vi "CTRE_PigeonIMU_GetYPR.vi"(8 "error in (no error)":errorcluster, 11 "PigeonIMUDevRef":T1={"DeviceStatus"={"status"=FALSE, "code"=0, "source"=""}, "Device Number"=0, "Type"=352321536, "Device ID"=0, "Handle"=0, "UsageFrame"=0, "Library Path"=path ""} {"Type" items=["CAN"=352321536, "TalonSRX"=33554432]}) -> (0 "error out":errorcluster, 2 "Yaw Pitch Roll":cluster{"Yaw":dbl, "Pitch":dbl, "Roll":dbl}, 3 "PigeonIMUDevRef":T1={"DeviceStatus"={"status"=FALSE, "code"=0, "source"=""}, "Device Number"=0, "Type"=352321536, "Device ID"=0, "Handle"=0, "UsageFrame"=0, "Library Path"=path ""} {"Type" items=["CAN"=352321536, "TalonSRX"=33554432]})   [LabVIEW 2016]
uses:
  <vilib>/Rock Robotics/WPI/ThirdParty/Sensors/Pigeon IMU/CTRE_PigeonIMU_DeviceRef.ctl
  <vilib>/Rock Robotics/WPI/ThirdParty/Sensors/Pigeon IMU/CTRE_PigeonIMU_ConnectionType.ctl
panel:
  out "error out 2":errorcluster
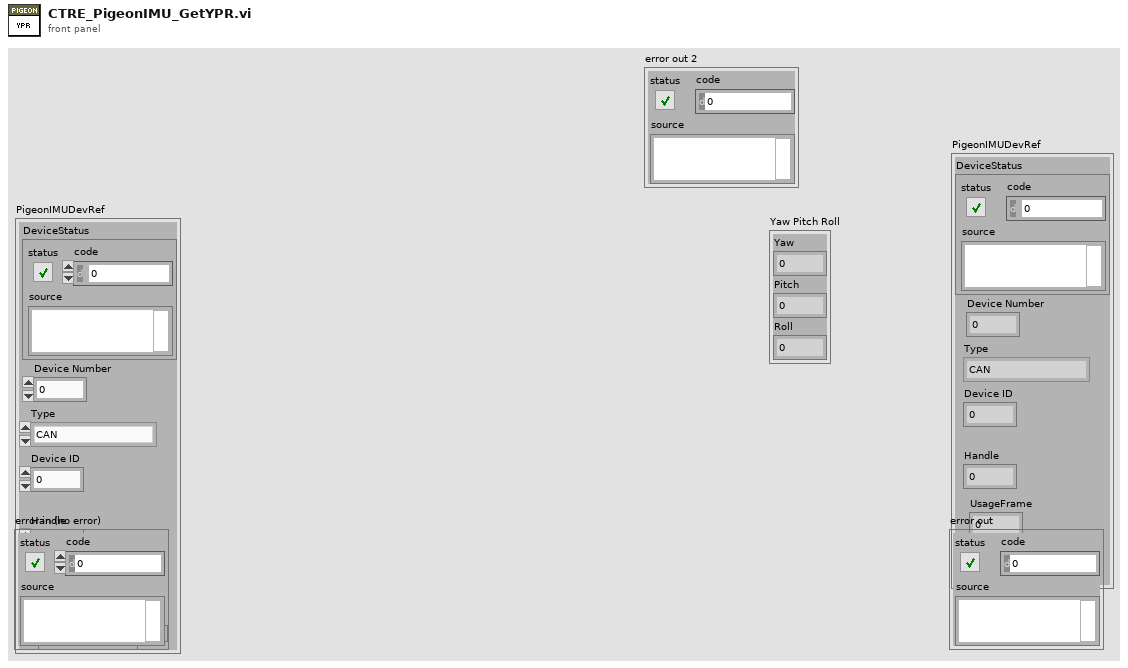
[diagram p1: front panel]
types:
  T1 = typedef "CTRE_PigeonIMU_DeviceRef.ctl" = cluster{"DeviceStatus":errorcluster, "Device Number":u8, "Type":T2, "Device ID":u32, "Handle":u64, "UsageFrame":u32, "Library Path":path}
  T2 = typedef "CTRE_PigeonIMU_ConnectionType.ctl" = u32
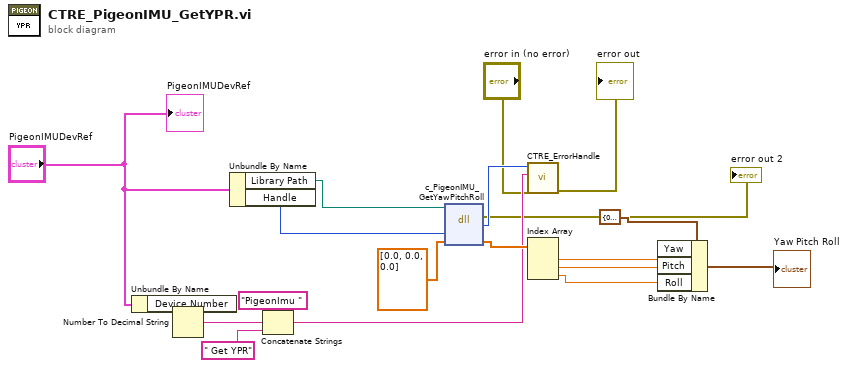
[diagram p0: block diagram]
diagram:
  n1 = Unbundle By Name("PigeonIMUDevRef") -> ("Device Number"=w10:u8)
  n2 = Number To Decimal String(number=w10) -> (decimal integer string=w9:string)  [unwired: 1 in]
  n3 = Unbundle By Name("PigeonIMUDevRef") -> ("Library Path"=w19:path, "Handle"=w18:u64)
  n4 = Concatenate Strings("PigeonImu " ("string"), w9, " Get YPR" ("string")) -> (w5:string)
  n5 = dll-call lib="?" fn="c_PigeonIMU_GetYawPitchRoll"(path in=w19, "handle"=w18, "ypr"=dbl[] [0.0, 0.0, 0.0]) -> (error out=→"error out 2":errorcluster, "return type"=w4:i32, "ypr"=w17:dbl[])  [unwired: 3 in, 1 out]
  n6 = call <vilib>:"CTRE_ErrorHandle.vi"("error in"="error in (no error)", "origin"=w5, "code"=w4) -> ("error out"=→"error out":errorcluster)  [unwired: 8 in]
  n7 = Index Array(array=w17) -> (element #1=w16:dbl, element #2=w15:dbl, element #3=w14:dbl)  [unwired: 3 in]
  n8 = Bundle By Name(cluster=cluster{"Yaw":dbl, "Pitch":dbl, "Roll":dbl} {"Yaw"=0.0, "Pitch"=0.0, "Roll"=0.0} ("YPR"), "Yaw"=w16, "Pitch"=w15, "Roll"=w14) -> (→"Yaw Pitch Roll":cluster{"Yaw":dbl, "Pitch":dbl, "Roll":dbl})
  "PigeonIMUDevRef" <- "PigeonIMUDevRef"
